vi "PRESENTASI GILMAN.vi"() -> ()   [LabVIEW 2017]
uses:
  <vilib>/Instr/_visa.llb/VISA Configure Serial Port (Instr).vi
panel:
  out "read buffer":string
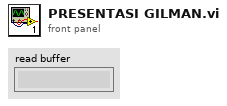
[diagram p1: front panel]
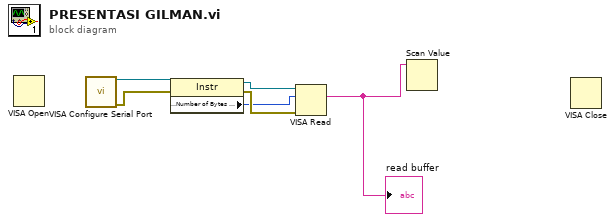
[diagram p0: block diagram]
diagram:
  n1 = VISA Open() -> ()  [unwired: 5 in, 2 out]
  n2 = call-poly "VISA Configure Serial Port"() -> ("VISA resource name out"=w6:refnum<visa-resource-name>, "error out"=w5:errorcluster)  [unwired: 14 in]
  n3 = property class="Instr"(reference=w6, error in=w5) -> (reference out=w4:refnum<visa-resource-name>, error out=w3:errorcluster, "Serial Settings:Number of Bytes at Serial Port"=w2:u32)
  n4 = VISA Read(VISA resource name=w4, byte count=w2, error in (no error)=w3) -> (read buffer=w1:string)  [unwired: 3 out]
  "read buffer" <- w1
  n5 = Scan Value(string=w1) -> ()  [unwired: 2 in, 2 out]
  n6 = VISA Close() -> ()  [unwired: 2 in, 1 out]
